vi "PSA Wait for Operation Complete (loop delay override).vi"(8 "error in (no error)":errorcluster, 9 "Maximum Time (10000ms)":i32=10000, 10 "loop delay (ms)":u32=1000, 11 "VISA resource name":refnum<visa-resource-name>) -> (0 "error out":errorcluster, 3 "VISA resource name out":refnum<visa-resource-name>)   [LabVIEW 2014]
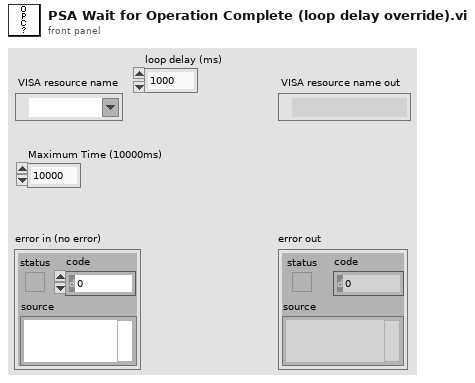
[diagram p1: front panel]
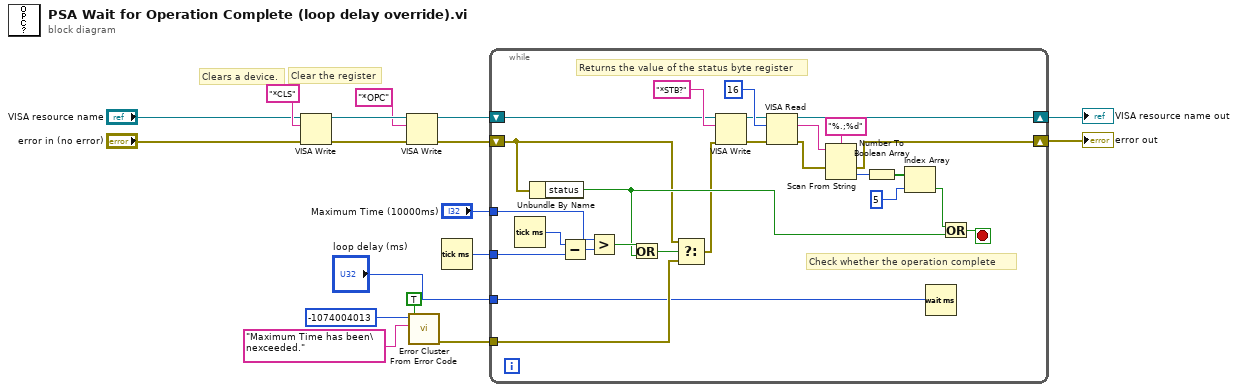
[diagram p0: block diagram]
diagram:
  # "Clears a device."
  # "Clear the register"
  n1 = VISA Write(VISA resource name="VISA resource name", write buffer="*CLS", error in (no error)="error in (no error)") -> (VISA resource name out=w7:refnum<visa-resource-name>, error out=w8:errorcluster)  [unwired: 1 out]
  n2 = VISA Write(VISA resource name=w7, write buffer="*OPC", error in (no error)=w8) -> (VISA resource name out=w6:refnum<visa-resource-name>, error out=w5:errorcluster)  [unwired: 1 out]
  n3 = call "Error Cluster From Error Code.vi"("show call chain? (False)"=TRUE, "error message (\"\")"="Maximum Time has been\nexceeded." ("error message (\"\")"), "error code (0)"=-1074004013) -> ("error out"=w11:errorcluster)  [unwired: 6 in]
  n4 = Tick Count (ms)() -> (millisecond timer value=w16:u32)
  n5 = while {
    tunnel: "Maximum Time (10000ms)" -> [w26]
    tunnel: w16 -> [w34]
    tunnel: w11 -> [w21]
    shift-right: [w32] -> w9
    shift-left: w5 -> [w19]
    shift-right: [w41] -> w10
    shift-left: w6 -> [w38]
    tunnel: "loop delay (ms)" -> [w18]
    stop <- w27 stop-if-true
    # "Check whether the operation complete"
    # "Returns the value of the status byte register"
    n6 = Tick Count (ms)() -> (millisecond timer value=w35:u32)
    n7 = Unbundle By Name(w19) -> ("status"=w22:bool)
    n8 = Subtract(x=w35, y=w34) -> (x-y=w25:u32)
    n9 = Greater?(x=w26, y=w25) -> (0:w24:bool)
    n10 = Or(x=w24, y=w22) -> (x .or. y?=w23:bool)
    n11 = Select(t=w19, s=w23, f=w21) -> (s? t:f=w20:errorcluster)
    n12 = VISA Write(VISA resource name=w38, write buffer="*STB?", error in (no error)=w20) -> (VISA resource name out=w36:refnum<visa-resource-name>, error out=w37:errorcluster)  [unwired: 1 out]
    n13 = VISA Read(VISA resource name=w36, byte count=u32 16, error in (no error)=w37) -> (VISA resource name out=w41:refnum<visa-resource-name>, read buffer=w43:string, error out=w33:errorcluster)  [unwired: 1 out]
    n14 = Scan From String(format string="%.;%d", input string=w43, error in=w33) -> (error out=w32:errorcluster, output 1=w29:i32)  [unwired: 2 in, 2 out]
    n15 = Number To Boolean Array(number=w29) -> (Boolean array=w30:bool[])
    n16 = Index Array(array=w30, index=5) -> (element=w28:bool)
    n17 = Wait (ms)(milliseconds to wait=w18) -> ()  [unwired: 1 out]
    n18 = Or(x=w28, y=w22) -> (x .or. y?=w27:bool)
  }
  "error out" <- w9
  "VISA resource name out" <- w10
